vi "Acquiring Data.vi"() -> ()   [LabVIEW 2015]
uses:
  <vilib>/express/express analysis/Spectral/Block/exnSpectralBlock spectral measurements peak poly.vi
  <vilib>/express/express analysis/Spectral/Block/exnSpectralBlock spectral measurements peak DDT.vi
  <vilib>/express/express analysis/Spectral/XNode/ExpressSpectralMeasurementsBlockNode.xnode
panel:
  in  "#Channels":i32=2
  in  "Device":u32
  out "Sound Waveform from Microphone":dynamicdata(graph)
  in  "Duration (s)":dbl=0.5
  in  "Sample rate (Hz)":dbl=22050.0
  in  "Resolution (bits)":i32=16
  in  "Stop":bool
  out "FFT Spectral Measurments":dynamicdata(graph)
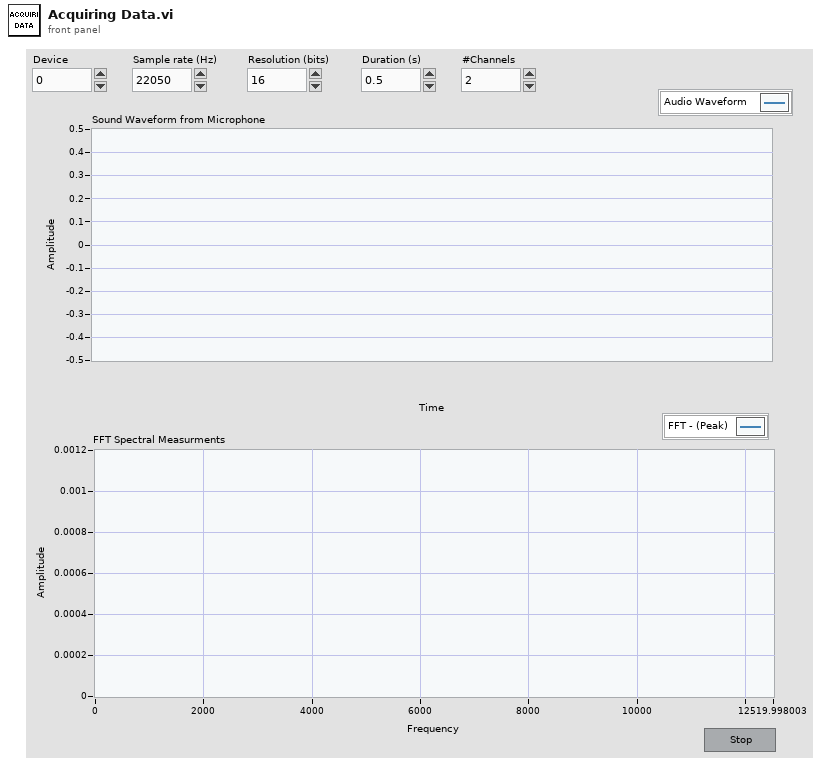
[diagram p1: front panel]
types:
  T1 = cluster{"averaging mode":u16, "weighting mode":u16, "number of averages":u32}
  T2 = cluster{"dB On (F)":bool, "unwrap phase (F)":bool, "convert to degree (F)":bool}
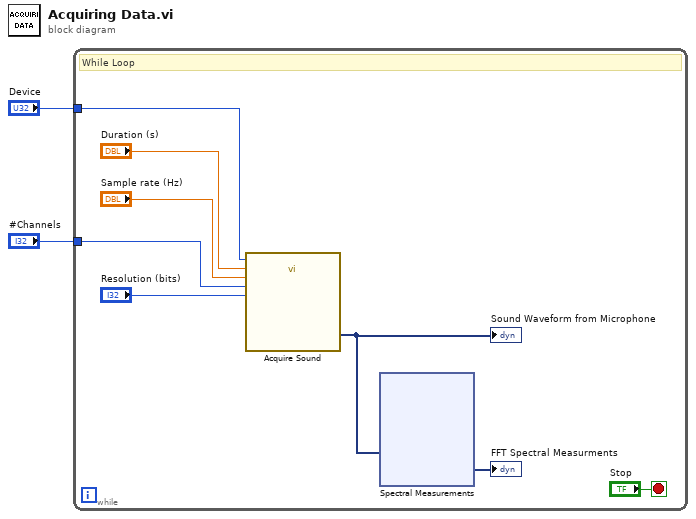
[diagram p0: block diagram]
diagram:
  n1 = while {
    tunnel: "Device" -> [w4]
    tunnel: "#Channels" -> [w3]
    stop <- "Stop" stop-if-true
    # "While Loop"
    n2 = call "Acquire Sound"("Device"=w4, "Duration (s)"="Duration (s)", "Sample rate (Hz)"="Sample rate (Hz)", "#Channels"=w3, "Resolution (bits)"="Resolution (bits)") -> ("Data"=w6:dynamicdata)  [unwired: 13 in, 1 out]
    "Sound Waveform from Microphone" <- w6
    n3 = xnode "Spectral Measurements"("Signals"=w6) -> ("FFT - (Peak)"=→"FFT Spectral Measurments":dynamicdata)  [unwired: 1 in, 2 out]
  }
